vi "Average Angle x8 (SubVI).vi"(9 "In Valid?":bool, 10 "Angle In":fxp<+/-,16,3> format="%.14g", 11 "End?":bool) -> (1 "Out Valid?":bool, 2 "Angle Out":fxp<+/-,16,3> format="%.14g", 3 "Done?":bool)   [LabVIEW 2015]
uses:
  Controls (FPGA)/Moving Average.ctl
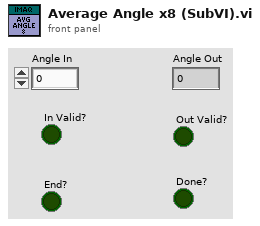
[diagram p1: front panel]
types:
  T1 = typedef "Moving Average.ctl" = enum16{"Enque", "Pass", "Deque"}
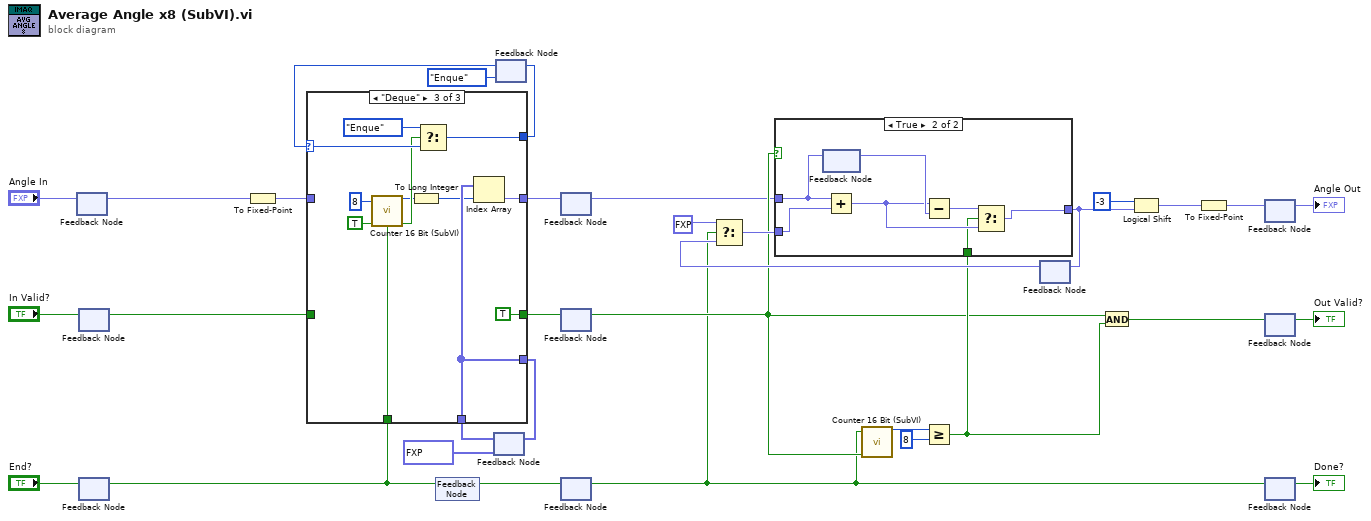
[diagram p0: block diagram]
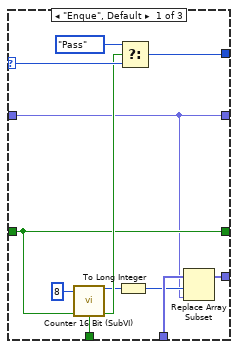
[diagram p2: hidden frame]
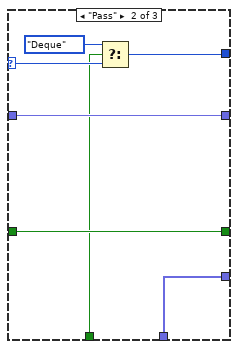
[diagram p3: hidden frame]
diagram:
  n1 = feedback-in #1("Angle In") -> ()
  n2 = feedback #1() -> (w1:fxp<+/-,16,3>)  [unwired: 1 in]
  n3 = feedback #2() -> (w8:bool)  [unwired: 1 in]
  n4 = feedback-in #2("In Valid?") -> ()
  n5 = feedback #3() -> (w19:bool)  [unwired: 1 in]
  n6 = feedback-in #3("End?") -> ()
  n7 = To Fixed-Point(number=w1) -> (fixed-point=w6:fxp<+/-,16,6>)  [unwired: 1 in]
  n8 = feedback-in #4(w19) -> ()
  n9 = feedback #4() -> (w13:bool)  [unwired: 1 in]
  n10 = feedback #5(fxp<+/-,16,6>[] [0.0, 0.0, 0.0, 0.0, 0.0, 0.0, 0.0, 0.0]) -> (w15:fxp<+/-,16,6>[])
  n11 = feedback #6(Moving_Average."Enque") -> (w21:T1)
  n12 = case shown="\"Deque\"" w21 {
    selector: w21 -> [w43 w48 w62]
    tunnel: [w42 w49 w61] -> w22
    tunnel: w8 -> [w39 w52 _]
    tunnel: w19 -> [w40 w47 w59]
    tunnel: w6 -> [w34 w51 _]
    tunnel: [w34 w51 w56] -> w17
    tunnel: [w39 w52 TRUE ("Boundary Valid? In")] -> w18
    tunnel: w15 -> [w38 w46 w58]
    tunnel: [w37 w46 w58] -> w14
    frame "Enque", Default {
      n13 = call "Counter 16 Bit (SubVI).vi"("Max. Count"=u16 8, "RESET"=w40, "Enable"=w39) -> ("Count"=w36:u16, "Count End?"=w41:bool)  [unwired: 10 in, 1 out]
      n14 = To Long Integer(number=w36) -> (32bit integer=w35:i32)
      n15 = Select(t=Moving_Average."Pass", s=w41, f=w43) -> (s? t:f=w42:T1)
      n16 = Replace Array Subset(array=w38, new element=w34, index=w35) -> (w37:fxp<+/-,16,6>[])
    }
    frame "Pass" {
      n17 = Select(t=Moving_Average."Deque", s=w47, f=w48) -> (s? t:f=w49:T1)
    }
    frame "Deque" {
      n18 = call "Counter 16 Bit (SubVI).vi"("Max. Count"=u16 8, "RESET"=w59, "Enable"=TRUE) -> ("Count"=w57:u16, "Count End?"=w60:bool)  [unwired: 10 in, 1 out]
      n19 = To Long Integer(number=w57) -> (32bit integer=w54:i32)
      n20 = Select(t=Moving_Average."Enque", s=w60, f=w62) -> (s? t:f=w61:T1)
      n21 = Index Array(array=w58, index=w54) -> (element=w56:fxp<+/-,16,6>)
    }
  }
  n22 = feedback-in #5(w14) -> ()
  n23 = feedback-in #6(w22) -> ()
  n24 = feedback-in #7(w17) -> ()
  n25 = feedback #7() -> (w5:fxp<+/-,16,6>)  [unwired: 1 in]
  n26 = feedback-in #8(w18) -> ()
  n27 = feedback #8() -> (w12:bool)  [unwired: 1 in]
  n28 = feedback-in #9(w13) -> ()
  n29 = feedback #9() -> (w11:bool)  [unwired: 1 in]
  n30 = call "Counter 16 Bit (SubVI).vi"("RESET"=w11, "Enable"=w12) -> ("Count"=w29:u16)  [unwired: 11 in, 2 out]
  n31 = Greater Or Equal?(x=w29, y=u16 8) -> (x >= y?=w23:bool)
  n32 = feedback #10() -> (w27:fxp<+/-,16,6>)  [unwired: 1 in]
  n33 = Select(t=fxp<+/-,16,6> 0.0, s=w11, f=w27) -> (s? t:f=w25:fxp<+/-,16,6>)
  n34 = case shown="True" w12 {
    tunnel: w5 -> [_ w66]
    tunnel: w23 -> [_ w69]
    tunnel: [w65 w68] -> w26
    tunnel: w25 -> [w65 w67]
    frame False {
    }
    frame True {
      n35 = feedback-in #11(w66) -> ()
      n36 = feedback #11() -> (w72:fxp<+/-,16,6>)  [unwired: 1 in]
      n37 = Add(x=w66, y=w67) -> (x+y=w70:fxp<+/-,16,6>)
      n38 = Subtract(x=w70, y=w72) -> (x-y=w71:fxp<+/-,16,6>)
      n39 = Select(t=w71, s=w69, f=w70) -> (s? t:f=w68:fxp<+/-,16,6>)
    }
  }
  n40 = feedback-in #10(w26) -> ()
  n41 = And(x=w12, y=w23) -> (x .and. y?=w24:bool)
  n42 = Logical Shift(y=i16 -3, x=w26) -> (x << y=w3:fxp<+/-,16,6>)
  n43 = To Fixed-Point(number=w3) -> (fixed-point=w2:fxp<+/-,16,3>)  [unwired: 1 in]
  n44 = feedback-in #12(w2) -> ()
  n45 = feedback #12() -> (→"Angle Out":fxp<+/-,16,3>)  [unwired: 1 in]
  n46 = feedback-in #13(w24) -> ()
  n47 = feedback #13() -> (→"Out Valid?":bool)  [unwired: 1 in]
  n48 = feedback-in #14(w11) -> ()
  n49 = feedback #14() -> (→"Done?":bool)  [unwired: 1 in]
